vi "CommonSig-Apply Ramp (2D).vi"(0 "Array in":dbl[][](array[numeric]), 5 "Ramp up (ms)":dbl=5.0, 7 "Ramp down (ms)":dbl=5.0, 9 "Fs (Hz)":dbl, 11 "error in (no error)":errorcluster, 12 "Asymmetric":bool) -> (4 "Array out":dbl[][](array[numeric]), 15 "error out":errorcluster)   [LabVIEW 2020]
uses:
  Classes/Gate/Shape.ctl
  Classes/Gate/Gate.lvclass/Gate.ctl
  00fa021d-ebe0-42e5-9c35-5538040c7da1.vi
  Classes/Gate/Write Ramp (ms).vi
  Classes/Gate/Write Down (ms).vi
  Classes/Gate/Write Asymmetric.vi
  Classes/Gate/Write Shape.vi
  Classes/Gate/Write Duration (ms).vi
  Classes/Gate/Gate.lvclass
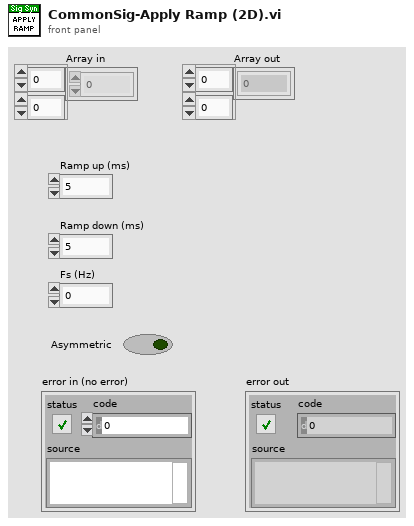
[diagram p1: front panel]
types:
  T1 = typedef "Gate.lvclass/Shape.ctl" = enum16{"OFF", "Rectangle", "Sine-squared", "Trapezoid"}
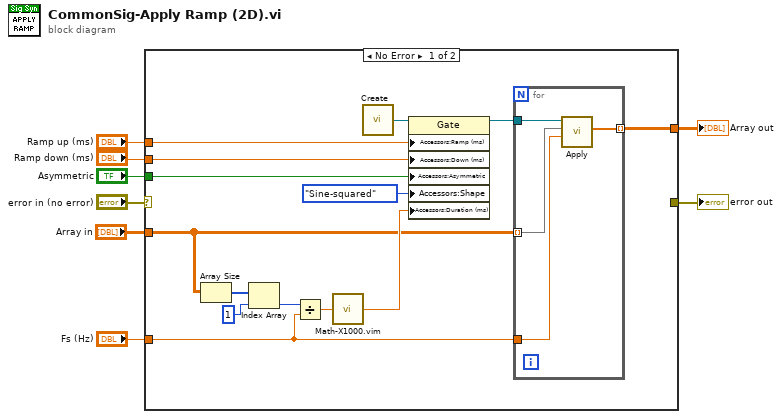
[diagram p0: block diagram]
diagram:
  n1 = case shown="No Error" "error in (no error)" {
    selector: "error in (no error)" -> [_ w27]
    tunnel: "Ramp up (ms)" -> [w22 _]
    tunnel: "Array in" -> [w9 w28]
    tunnel: [w18 w28] -> w6
    tunnel: "Fs (Hz)" -> [w19 _]
    tunnel: "Ramp down (ms)" -> [w21 _]
    tunnel: "Asymmetric" -> [w20 _]
    tunnel: [_ w27] -> w1
    frame No Error {
      n2 = Array Size(array=w9) -> (size(s)=w14:i32[])
      n3 = Index Array(array=w14, index=1) -> (element=w12:i32)
      n4 = Divide(x=w12, y=w19) -> (x/y=w11:dbl)
      n5 = call "Math-X1000.vim"("X"=w11) -> ("1000X"=w10:dbl)
      n6 = call "Create.vi"() -> ("Gate"=w17:refnum<class "Gate.lvclass">)  [unwired: 15 in]
      n7 = property class="Gate"(reference=w17, "Accessors:Ramp (ms)"=w22, "Accessors:Down (ms)"=w21, "Accessors:Asymmetric"=w20, "Accessors:Shape"=Shape."Sine-squared" ("Shape"), "Accessors:Duration (ms)"=w10) -> (reference out=w16:refnum<class "Gate.lvclass">)  [unwired: 1 in, 1 out]
      n8 = for {
        tunnel: w16 -> [w26]
        tunnel: w9 -> [w25] mode=indexing
        tunnel: [w24] -> w18 mode=indexing
        tunnel: w19 -> [w23]
        n9 = call "Apply.vi"("Fs (Hz)"=w23, "Array in"=w25, "Gate in"=w26) -> ("Array out"=w24:dbl[])  [unwired: 6 in, 2 out]
      }
    }
    frame Error {
    }
  }
  "Array out" <- w6
  "error out" <- w1
